vi "Subvi PMT simulator.vi"(9 "PulseSequence":bool[](array[boolean])=[FALSE, FALSE, FALSE, FALSE, FALSE, FALSE, FALSE, FALSE, FALSE, FALSE, FALSE, FALSE, FALSE, FALSE, FALSE, FALSE, FALSE, FALSE, FALSE, FALSE], 11 "nPulses":u8) -> (1 "Output":bool)   [LabVIEW 2017]
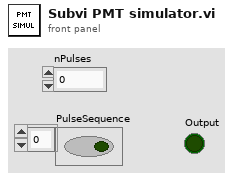
[diagram p1: front panel]
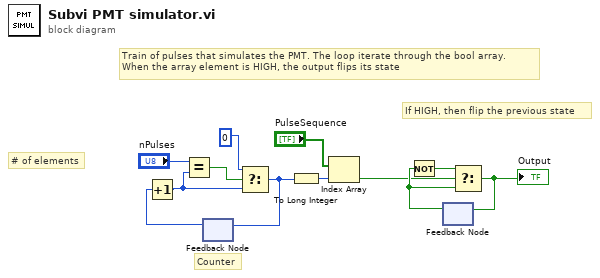
[diagram p0: block diagram]
diagram:
  # "Counter"
  # "If HIGH, then flip the previous state"
  # "# of elements"
  # "Train of pulses that simulates the PMT. The loop iterate through the bool array.\nWhen the array element is HIGH, the output flips its state"
  n1 = feedback #1() -> (w3:u8)  [unwired: 1 in]
  n2 = Increment(x=w3) -> (x+1=w4:u8)
  n3 = Equal?(x="nPulses", y=w4) -> (x = y?=w7:bool)
  n4 = Select(t=u8 0, s=w7, f=w4) -> (s? t:f=w5:u8)
  n5 = feedback-in #1(w5) -> ()
  n6 = To Long Integer(number=w5) -> (32bit integer=w6:i32)
  n7 = Index Array(array="PulseSequence", index=w6) -> (element=w10:bool)
  n8 = feedback #2() -> (w12:bool)  [unwired: 1 in]
  n9 = Not(x=w12) -> (.not. x?=w11:bool)
  n10 = Select(t=w11, s=w10, f=w12) -> (s? t:f=w2:bool)
  "Output" <- w2
  n11 = feedback-in #2(w2) -> ()
